vi "QUDI_QPD_laser_control.vi"() -> ()   [LabVIEW 2015]
uses:
  <vilib>/Platform/TimedLoop/XDataNode/timing_clust.ctl
  <vilib>/Platform/TimedLoop/XDataNode/nitl_modes.ctl
  <vilib>/Platform/TimedLoop/XDataNode/wakeup.ctl
  <vilib>/rvi/FXPMathLib/basic elements/FxpIntAccumulator/subVIs/nifxpmath_IntAccumulator_SimConfig.ctl
  <vilib>/rvi/Emulation/niFpgaGetClockAttributes.vi
  <vilib>/rvi/Emulation/niFpgaSctlEmulationGetInTimedLoop.vi
  <vilib>/rvi/Emulation/niFpgaEmulationReportErrorSimple.vi
  <vilib>/rvi/Emulation/niFpgaProcessEmulError.vi
  <vilib>/rvi/eio/common/nirviEmuTemplateMethod_errors.vi
  <vilib>/rvi/Analysis/common/codeGenErrors/XNode/niFpgaXNodeCodeGenErrorHandle.vi
  <vilib>/rvi/Emulation/niFpgaCriticalErrorInLSC.vi
  <vilib>/rvi/FXPMathLib/basic elements/FxpIntAccumulator/simVIs/DllFxpIntAccumulator_sub.vi
  <vilib>/eio/EIONode/EIONode.xnode
  <vilib>/rvi/Analysis/measure/dc-rms/XNode/niFpgaDC-RMS.xnode
  <vilib>/Platform/TimedLoop/XDataNode/XDataNode.xnode
  <vilib>/rvi/FXPMathLib/basic elements/FxpIntAccumulator/XNode/nifxpmath_IntAccumulator.xnode
  <vilib>/Platform/TimedLoop/XDataNode/XDNodeRunTimeDep.lvlib
panel:
  out "counter":u32
  out "I":i16
  out "Y":i16
  out "X":i16
  in  "561":i16
  in  "640":i16
  in  "405":i16
  in  "488":i16
  in  "integration_time_us":u32=100 caption="Count(uSec)"
  in  "stop":bool
  out "duration_ms":u32
  in  "reset_counter":bool
  in  "Update lasers":bool
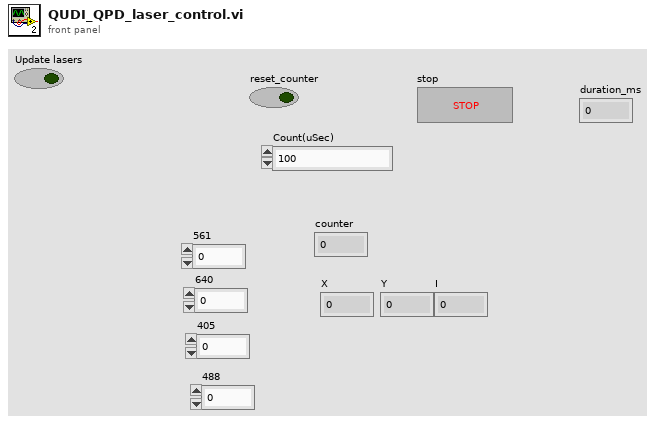
[diagram p1: front panel]
types:
  T1 = typedef "XDNodeRunTimeDep.lvlib/timing_clust.ctl" = cluster{"Expected End [f-1]":u64, "Actual End [f-1]":u64, "Finished Late? [f-1]":bool, "Expected End [i-1]":u64, "Actual End [i-1]":u64, "Finished Late? [i-1]":bool, "Expected Start [i]":u64, "Actual Start [i]":u64, "Expected Start [f]":u64, "Actual Start [f]":u64, "Source Name":string, "Structure Name":string, "Period":i64, "Deadline":i64, "Offset":i64, "Start":i64, "Priority":i32, "Timeout":i32, "Mode":T2, "Wakeup Reason":T3, "Error":errorcluster, "Source Type":string, "Secondary Source Type":string, "Global End Time":u64, "Global Start Time":u64, "Frame Duration":u64, "Iteration Duration":u64, "Assigned CPU":i32, "I/O Scan Engine Mode":u32}
  T2 = typedef "XDNodeRunTimeDep.lvlib/nitl_modes.ctl" = enum32{"No Change", "Process missed periods, maintain original phase", "Discard missed periods, maintain original phase", "Process missed periods, ignore original phase", "Discard missed periods, ignore original phase"}
  T3 = typedef "XDNodeRunTimeDep.lvlib/wakeup.ctl" = enum32{"Normal", "Aborted", "Asynchronous wakeup", "Timing source error", "Timed loop error", "Timeout"}
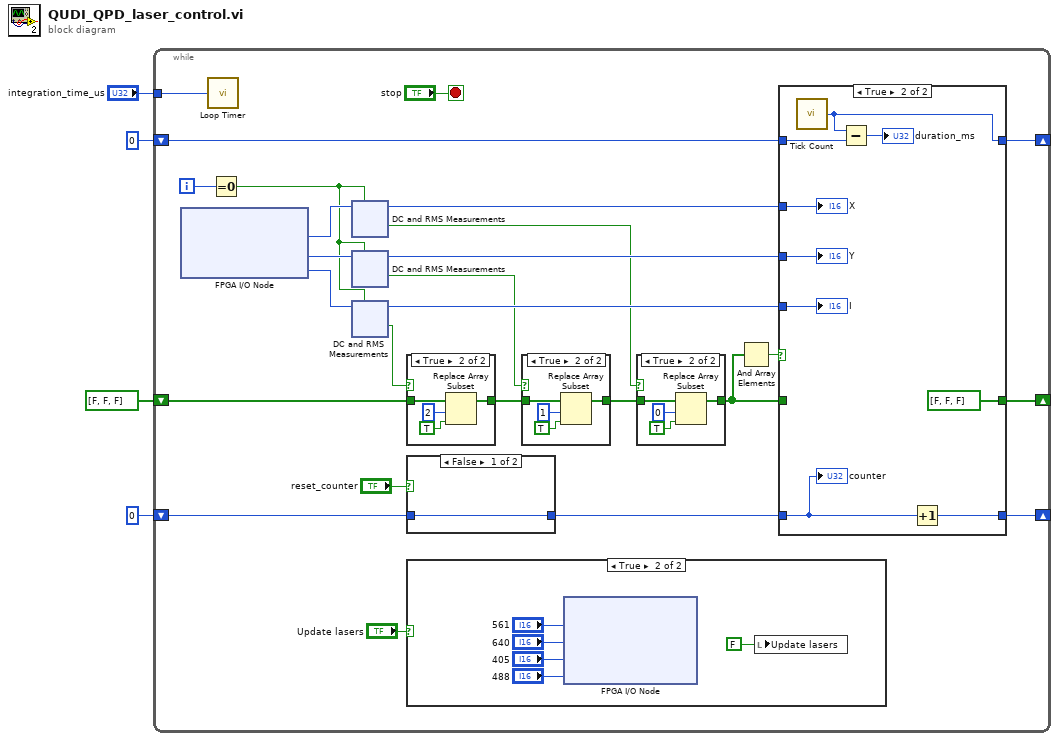
[diagram p0: block diagram]
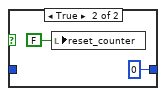
[diagram p3: hidden frame]
diagram:
  n1 = while {
    shift-right: [w13] -> _
    shift-left: bool[] [FALSE, FALSE, FALSE] ("initialized array") -> [w21]
    shift-right: [w11] -> _
    shift-left: u32 0 -> [w12]
    tunnel: "integration_time_us" -> [w10]
    shift-right: [w9] -> _
    shift-left: u32 0 -> [w7]
    i -> [w28]
    stop <- "stop" stop-if-true
    n2 = xnode "FPGA I/O Node"() -> ("Connector0/AI0"=w30:i16, "Connector0/AI1"=w26:i16, "Connector0/AI2"=w25:i16)  [unwired: 3 in, 3 out]
    n3 = call "Loop Timer"("Count(uSec)"=w10) -> ()  [unwired: 1 out]
    n4 = Equal To 0?(x=w28) -> (x = 0?=w22:bool)
    n5 = xnode "DC and RMS Measurements"("input data"=w30, "reset"=w22) -> ("DC"=w27:i16, "output valid"=w16:bool)
    n6 = xnode "DC and RMS Measurements"("input data"=w26, "reset"=w22) -> ("DC"=w24:i16, "output valid"=w17:bool)
    n7 = xnode "DC and RMS Measurements"("input data"=w25, "reset"=w22) -> ("DC"=w23:i16, "output valid"=w18:bool)
    n8 = case shown="True" w18 {
      tunnel: w21 -> [w44 w47]
      tunnel: [w44 w45] -> w20
      frame False {
      }
      frame True {
        n9 = Replace Array Subset(array=w47, new element=TRUE, index=2) -> (w45:bool[])
      }
    }
    n10 = case shown="False" "reset_counter" {
      tunnel: w7 -> [w36 _]
      tunnel: [w36 u32 0] -> w6
      frame False {
      }
      frame True {
        n11 = local write "reset_counter"(FALSE ("Reset counter")) -> ()
      }
    }
    n12 = case shown="True" "Update lasers" {
      frame False {
      }
      frame True {
        n13 = xnode "FPGA I/O Node"("Connector0/AO0"="561", "Connector0/AO1"="640", "Connector0/AO2"="405", "Connector0/AO3"="488") -> ()  [unwired: 4 in, 4 out]
        n14 = local write "Update lasers"(FALSE ("Update lasers")) -> ()
      }
    }
    n15 = case shown="True" w17 {
      tunnel: w20 -> [w49 w52]
      tunnel: [w49 w50] -> w19
      frame False {
      }
      frame True {
        n16 = Replace Array Subset(array=w52, new element=TRUE, index=1) -> (w50:bool[])
      }
    }
    n17 = case shown="True" w16 {
      tunnel: [w39 w41] -> w14
      tunnel: w19 -> [w39 w40]
      frame False {
      }
      frame True {
        n18 = Replace Array Subset(array=w40, new element=TRUE, index=0) -> (w41:bool[])
      }
    }
    n19 = And Array Elements(Boolean array=w14) -> (logical AND=w15:bool)
    n20 = case shown="True" w15 {
      tunnel: w27 -> [_ w60]
      tunnel: w24 -> [_ w59]
      tunnel: w23 -> [_ w58]
      tunnel: w14 -> [w56 _]
      tunnel: [w56 bool[] [FALSE, FALSE, FALSE] ("initialized array")] -> w13
      tunnel: w12 -> [w55 w64]
      tunnel: [w55 w62] -> w11
      tunnel: w6 -> [w54 w57]
      tunnel: [w54 w61] -> w9
      frame False {
      }
      frame True {
        n21 = call "Tick Count"() -> ("Tick Count(mSec)"=w62:u32)
        n22 = Subtract(x=w62, y=w64) -> (x-y=→"duration_ms":u32)
        n23 = Increment(x=w57) -> (x+1=w61:u32)
        "X" <- w60
        "Y" <- w59
        "I" <- w58
        "counter" <- w57
      }
    }
  }
